vi "Synced Example.vi"() -> ()   [LabVIEW 2020, in "2D Array Example.lvlib"]
uses:
  2D Array Example.lvlib
  OOPanel/2DArrayManager/Direction.ctl
  ExBlank/ExBlank.lvclass
  C:/dev/lv20CE/lv-oopanel/OOPanel/2DPanelBlank/2DPanelBlank.lvclass
  2DArrayPanel/2DArrayPanel.lvclass
  C:/dev/lv20CE/lv-oopanel/OOPanel/ArrayPanel/ArrayPanel.lvclass
  OOPanel/2DArrayManager/2DArrayManager.lvclass
panel:
  out "error out":errorcluster
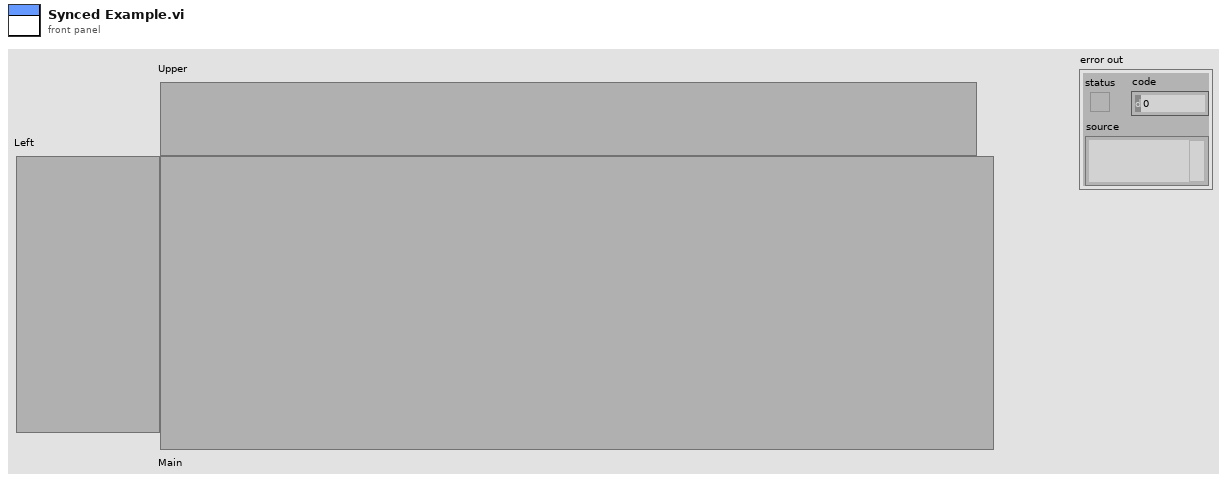
[diagram p1: front panel]
types:
  T1 = typedef "OOPanel.lvlib/2DArrayManager.lvclass/Direction.ctl" = enum16{"Vertical", "Horizontal", "Both"}
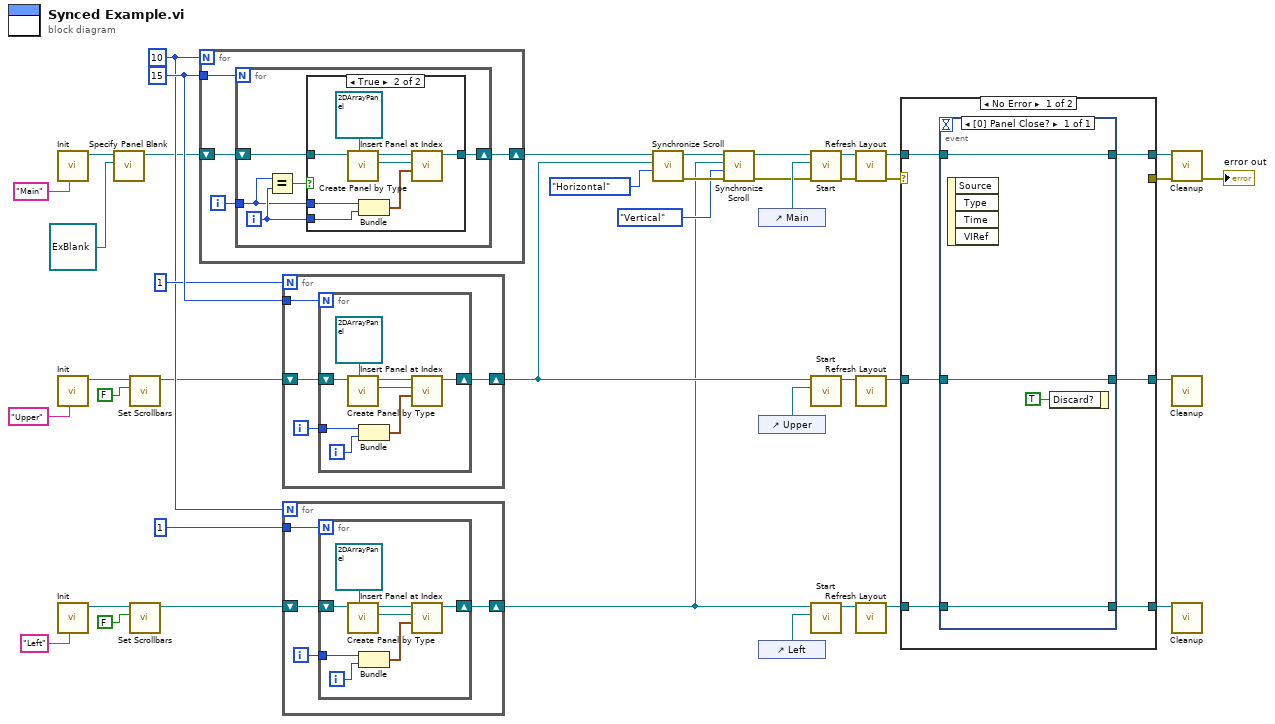
[diagram p0: block diagram]
diagram:
  w33 = 15
  w30 = 10
  n1 = call "Init.vi"("Name (Caller VI)"="Main") -> ("2DArrayManager out"=w36:refnum<class "2DArrayManager.lvclass">)  [unwired: 9 in, 1 out]
  n2 = call "Init.vi"("Name (Caller VI)"="Upper") -> ("2DArrayManager out"=w35:refnum<class "2DArrayManager.lvclass">)  [unwired: 9 in, 1 out]
  n3 = call "Init.vi"("Name (Caller VI)"="Left") -> ("2DArrayManager out"=w34:refnum<class "2DArrayManager.lvclass">)  [unwired: 9 in, 1 out]
  n4 = call "Specify Panel Blank.vi"("Blank VI"=refnum<class "ExBlank.lvclass"> refnum ("2D Array Example.lvlib:ExBlank.lvclass"), "2DArrayManager in"=w36) -> ("2DArrayManager out"=w5:refnum<class "2DArrayManager.lvclass">)  [unwired: 8 in, 1 out]
  n5 = call "Set Scrollbars.vi"("Scrollbars"=FALSE, "2DArrayManager in"=w35) -> ("2DArrayManager out"=w9:refnum<class "2DArrayManager.lvclass">)  [unwired: 8 in, 1 out]
  n6 = call "Set Scrollbars.vi"("Scrollbars"=FALSE, "2DArrayManager in"=w34) -> ("2DArrayManager out"=w8:refnum<class "2DArrayManager.lvclass">)  [unwired: 8 in, 1 out]
  n7 = for {
    N: w30 -> [_]
    tunnel: w33 -> [w45]
    shift-right: [w43] -> w29
    shift-left: w5 -> [w44]
    i -> [w42]
    n8 = for {
      N: w45 -> [_]
      shift-right: [w49] -> w43
      shift-left: w44 -> [w50]
      tunnel: w42 -> [w47]
      i -> [w48]
      n9 = Equal?(x=w47, y=w48) -> (x = y?=w46:bool)
      n10 = case shown="True" w46 {
        tunnel: w50 -> [w51 w59]
        tunnel: [w51 w54] -> w49
        tunnel: w48 -> [_ w53]
        tunnel: w47 -> [_ w52]
        frame False {
        }
        frame True {
          n11 = call "Create Panel by Type.vi"("Panel Type"=refnum<class "2DArrayPanel.lvclass"> refnum ("2D Array Example.lvlib:2DArrayPanel.lvclass"), "2DArrayManager in"=w59) -> ("Panel"=w56:refnum<class "2DArrayPanel.lvclass">, "2DArrayManager out"=w57:refnum<class "2DArrayManager.lvclass">)  [unwired: 7 in, 1 out]
          n12 = Bundle(w52, w53) -> (w55:cluster{i32, i32})  [unwired: 1 in]
          n13 = call "Insert Panel at Index.vi"("2D Index"=w55, "ArrayPanel"=w56, "2DArrayManager in"=w57) -> ("2DArrayManager out"=w54:refnum<class "2DArrayManager.lvclass">)  [unwired: 5 in, 3 out]
        }
      }
    }
  }
  n14 = for {
    N: 1 -> [_]
    tunnel: w33 -> [w63]
    shift-right: [w61] -> w24
    shift-left: w9 -> [w62]
    i -> [w60]
    n15 = for {
      N: w63 -> [_]
      shift-right: [w64] -> w61
      shift-left: w62 -> [w69]
      tunnel: w60 -> [w71]
      i -> [w70]
      n16 = call "Create Panel by Type.vi"("Panel Type"=refnum<class "2DArrayPanel.lvclass"> refnum ("2D Array Example.lvlib:2DArrayPanel.lvclass"), "2DArrayManager in"=w69) -> ("Panel"=w66:refnum<class "2DArrayPanel.lvclass">, "2DArrayManager out"=w67:refnum<class "2DArrayManager.lvclass">)  [unwired: 7 in, 1 out]
      n17 = Bundle(w71, w70) -> (w65:cluster{i32, i32})  [unwired: 1 in]
      n18 = call "Insert Panel at Index.vi"("2D Index"=w65, "ArrayPanel"=w66, "2DArrayManager in"=w67) -> ("2DArrayManager out"=w64:refnum<class "2DArrayManager.lvclass">)  [unwired: 5 in, 3 out]
    }
  }
  n19 = for {
    N: w30 -> [_]
    tunnel: 1 -> [w75]
    shift-right: [w73] -> w1
    shift-left: w8 -> [w74]
    i -> [w72]
    n20 = for {
      N: w75 -> [_]
      shift-right: [w76] -> w73
      shift-left: w74 -> [w81]
      tunnel: w72 -> [w83]
      i -> [w82]
      n21 = call "Create Panel by Type.vi"("Panel Type"=refnum<class "2DArrayPanel.lvclass"> refnum ("2D Array Example.lvlib:2DArrayPanel.lvclass"), "2DArrayManager in"=w81) -> ("Panel"=w78:refnum<class "2DArrayPanel.lvclass">, "2DArrayManager out"=w79:refnum<class "2DArrayManager.lvclass">)  [unwired: 7 in, 1 out]
      n22 = Bundle(w83, w82) -> (w77:cluster{i32, i32})  [unwired: 1 in]
      n23 = call "Insert Panel at Index.vi"("2D Index"=w77, "ArrayPanel"=w78, "2DArrayManager in"=w79) -> ("2DArrayManager out"=w76:refnum<class "2DArrayManager.lvclass">)  [unwired: 5 in, 3 out]
    }
  }
  n24 = call "Synchronize Scroll.vi"("Direction"=Direction."Horizontal", "Other 2D Array"=w24, "2DArrayManager in"=w29) -> ("error out"=w40:errorcluster, "2DArrayManager out"=w27:refnum<class "2DArrayManager.lvclass">)  [unwired: 7 in]
  n25 = call "Synchronize Scroll.vi"("error in (no error)"=w40, "Direction"=Direction."Vertical", "Other 2D Array"=w1, "2DArrayManager in"=w27) -> ("error out"=w18:errorcluster, "2DArrayManager out"=w3:refnum<class "2DArrayManager.lvclass">)  [unwired: 6 in]
  n26 = control-ref of="Main"() -> (w25:refnum<vi>)
  n27 = control-ref of="Upper"() -> (w23:refnum<vi>)
  n28 = control-ref of="Left"() -> (w22:refnum<vi>)
  n29 = call "Start.vi"("error in (no error)"=w18, "Container"=w25, "2DArrayManager in"=w3) -> ("error out"=w2:errorcluster, "2DArrayManager out"=w19:refnum<class "2DArrayManager.lvclass">)  [unwired: 7 in]
  n30 = call "Start.vi"("Container"=w23, "2DArrayManager in"=w24) -> ("2DArrayManager out"=w20:refnum<class "2DArrayManager.lvclass">)  [unwired: 8 in, 1 out]
  n31 = call "Start.vi"("Container"=w22, "2DArrayManager in"=w1) -> ("2DArrayManager out"=w21:refnum<class "2DArrayManager.lvclass">)  [unwired: 8 in, 1 out]
  n32 = call "Refresh Layout.vi"("error in (no error)"=w2, "2DArrayManager in"=w19) -> ("error out"=w17:errorcluster, "2DArrayManager out"=w16:refnum<class "2DArrayManager.lvclass">)  [unwired: 8 in]
  n33 = call "Refresh Layout.vi"("2DArrayManager in"=w20) -> ("2DArrayManager out"=w15:refnum<class "2DArrayManager.lvclass">)  [unwired: 9 in, 1 out]
  n34 = call "Refresh Layout.vi"("2DArrayManager in"=w21) -> ("2DArrayManager out"=w14:refnum<class "2DArrayManager.lvclass">)  [unwired: 9 in, 1 out]
  n35 = case shown="No Error" w17 {
    selector: w17 -> [_ w94]
    tunnel: w16 -> [w84 w97]
    tunnel: w15 -> [w86 w96]
    tunnel: w14 -> [w88 w95]
    tunnel: [w89 w95] -> w12
    tunnel: [w87 w96] -> w11
    tunnel: [w85 w97] -> w13
    tunnel: [_ w94] -> w10
    frame No Error {
      n36 = event shown="[0] Panel Close?" {
        selector: _ -> [_]
        dyn-events: _ -> [_]
        timeout: _ -> [_]
        tunnel: [w93] -> w89
        tunnel: w88 -> [w93]
        tunnel: [w92] -> w87
        tunnel: w86 -> [w92]
        tunnel: [w91] -> w85
        tunnel: w84 -> [w91]
        event Panel Close? {
          n37 = event-data() -> ()  [unwired: 1 in, 4 out]
          n38 = event-data("Discard?"=TRUE) -> ()  [unwired: 1 in, 1 out]
        }
      }
    }
    frame Error {
    }
  }
  n39 = call "Cleanup.vi"("error in (no error)"=w10, "2DArrayManager in"=w13) -> ("error out"=→"error out":errorcluster)  [unwired: 9 in]
  n40 = call "Cleanup.vi"("2DArrayManager in"=w11) -> ()  [unwired: 10 in, 1 out]
  n41 = call "Cleanup.vi"("2DArrayManager in"=w12) -> ()  [unwired: 10 in, 1 out]
